vi "start.vi"(8 "error in (no error)":errorcluster caption="错误输入（无错误）", 10 "strPartNo":string, 11 "EEPromCodeService 引用句柄":refnum<k24>) -> (0 "error out":errorcluster caption="错误输出", 2 ".NET:EEPromCodeService.ParaClass":T1, 3 "EEPromCodeService 引用句柄输出":refnum<k24>)   [LabVIEW 2011]
uses:
  Data/EEPromCodeService.dll
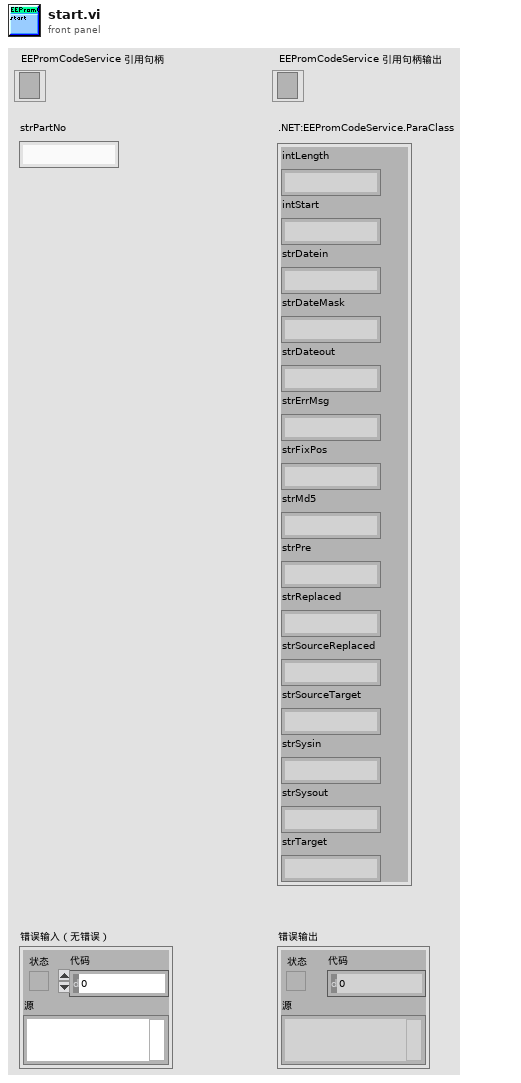
[diagram p1: front panel]
types:
  T1 = cluster{"intLength":string, "intStart":string, "strDatein":string, "strDateMask":string, "strDateout":string, "strErrMsg":string, "strFixPos":string, "strMd5":string, "strPre":string, "strReplaced":string, "strSourceReplaced":string, "strSourceTarget":string, "strSysin":string, "strSysout":string, "strTarget":string}
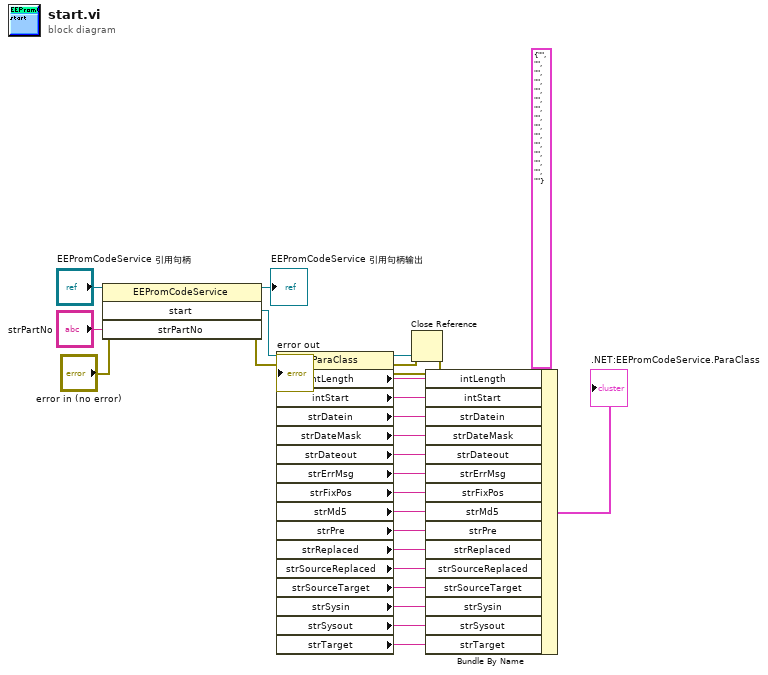
[diagram p0: block diagram]
diagram:
  n1 = invoke class="EEPromCodeService" method="start"(reference="EEPromCodeService 引用句柄", error in="error in (no error)", "strPartNo"="strPartNo") -> (reference out=→"EEPromCodeService 引用句柄输出":refnum<k24>, error out=w4:errorcluster, "start"=w23:refnum<k24>)  [unwired: 1 in, 1 out]
  n2 = property class="ParaClass"(reference=w23, error in=w4) -> (reference out=w3:refnum<k24>, error out=w2:errorcluster, "intLength"=w20:string, "intStart"=w19:string, "strDatein"=w18:string, "strDateMask"=w17:string, "strDateout"=w16:string, "strErrMsg"=w15:string, "strFixPos"=w14:string, "strMd5"=w13:string, "strPre"=w12:string, "strReplaced"=w11:string, "strSourceReplaced"=w10:string, "strSourceTarget"=w9:string, "strSysin"=w8:string, "strSysout"=w7:string, "strTarget"=w6:string)
  n3 = Close Reference(reference=w3, error in (no error)=w2) -> (error out=→"error out":errorcluster)
  n4 = Bundle By Name(cluster=T1 {"intLength"="", "intStart"="", "strDatein"="", "strDateMask"="", "strDateout"="", "strErrMsg"="", "strFixPos"="", "strMd5"="", "strPre"="", "strReplaced"="", "strSourceReplaced"="", "strSourceTarget"="", "strSysin"="", "strSysout"="", "strTarget"=""} (".NET:EEPromCodeService.ParaClass"), "intLength"=w20, "intStart"=w19, "strDatein"=w18, "strDateMask"=w17, "strDateout"=w16, "strErrMsg"=w15, "strFixPos"=w14, "strMd5"=w13, "strPre"=w12, "strReplaced"=w11, "strSourceReplaced"=w10, "strSourceTarget"=w9, "strSysin"=w8, "strSysout"=w7, "strTarget"=w6) -> (→".NET:EEPromCodeService.ParaClass":T1)
